vi "Measure.vi"(6 "error in (no error)":errorcluster, 9 "Generic Data Acquisition in":refnum<class "Generic Data Acquisition.lvclass">) -> (0 "error out":errorcluster, 2 "Array of Measurement":dbl[](array[numeric]), 3 "Generic Data Acquisition out":refnum<class "Generic Data Acquisition.lvclass">)   [LabVIEW 2014, in "Generic Data Acquisition.lvlib" / "Generic Data Acquisition.lvclass"]
uses:
  Generic Data Acquisition.lvclass
  Abstract Sensor/Abstract Sensor.lvclass
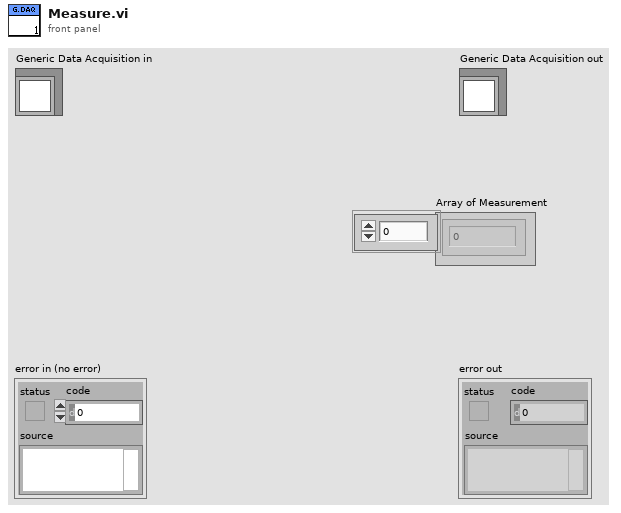
[diagram p1: front panel]
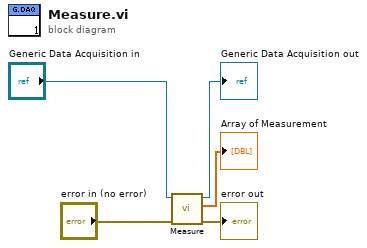
[diagram p0: block diagram]
diagram:
  n1 = call-parent "Measure.vi"("error in (no error)"="error in (no error)", "Abstract Sensor in"="Generic Data Acquisition in") -> ("error out"=→"error out":errorcluster, "Array of Measurement"=→"Array of Measurement":dbl[], "Abstract Sensor out"=→"Generic Data Acquisition out":refnum<class "Generic Data Acquisition.lvclass">)  [unwired: 5 in]
